vi "Read VI Path.vi"(8 "error in (no error)":errorcluster, 11 "VI in":refnum<class "VI.lvclass">) -> (0 "error out":errorcluster, 2 "VI Path":path, 3 "VI out":refnum<class "VI.lvclass">)   [LabVIEW 2019, in "Panther Dashboard.lvlib" / "VI.lvclass"]
uses:
  VI.lvclass
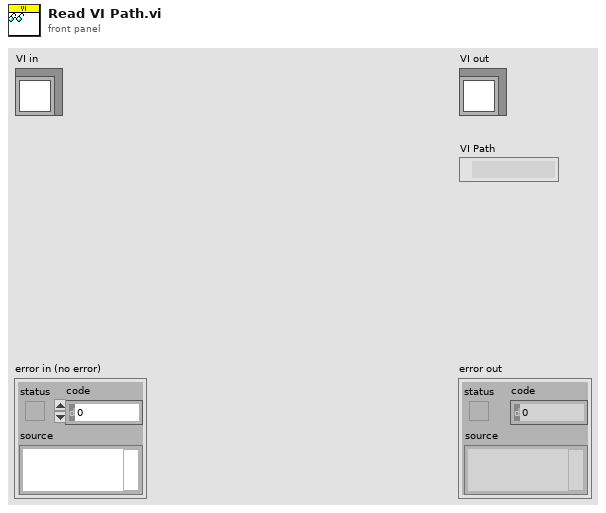
[diagram p1: front panel]
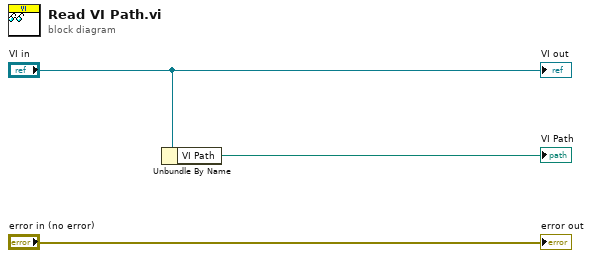
[diagram p0: block diagram]
diagram:
  n1 = Unbundle By Name("VI in") -> ("VI Path"=→"VI Path":path)
  "error out" <- "error in (no error)"
  "VI out" <- "VI in"
